vi "图像色彩识别.vi"() -> ()   [LabVIEW 2020]
uses:
  <vilib>/vision/NI_Vision_Development_Module.lvlib
panel:
  out "FoundYellow":bool
  out "FoundGreen":bool
  out "error out":errorcluster
  out "FoundRed":bool
  in  "停止":bool
  out "Color Spectrum":dbl[](array[numeric]) format="%.2f"
  in  "Rectangle":T1={"Left"=300, "Top"=170, "Right"=441, "Bottom"=320, "Rotation"=0.0} {"Rotation" min=-90.0 max=90.0 step=1.0 format="%.2f"; "Left" scale=0.0..1024.0; "Right" scale=0.0..1024.0}
  in  "File Path":path
  out "Image":T2(plugin-control)
  # "画框给出的左边值x,y格式给\n出，输入时注意对应"
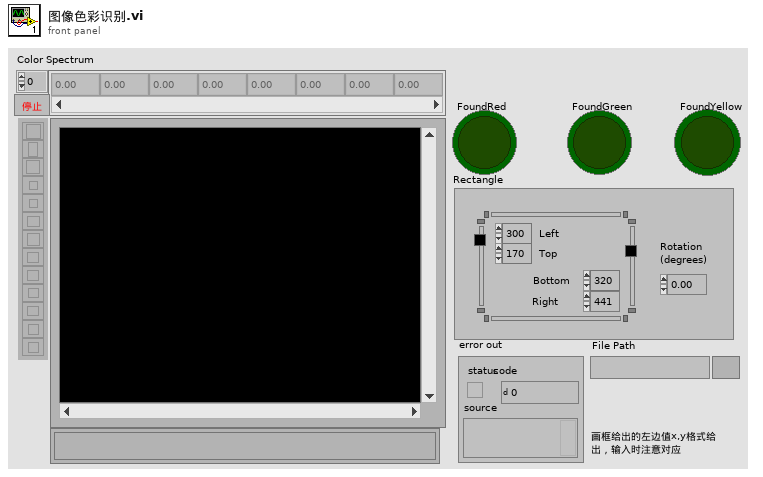
[diagram p1: front panel]
types:
  T1 = typedef "IMAQ Rectangle" = cluster{"Left":i32, "Top":i32, "Right":i32, "Bottom":i32, "Rotation":dbl}
  T2 = typedef "IMAQ Image.ctl" = refnum<image>
  T3 = typedef "ROI Descriptor" = cluster{"Global Rectangle":i32[], "Contours":cluster{"ID":enum32{"External", "Internal"}, "Type":u32, "Coordinates":i32[]}[]}
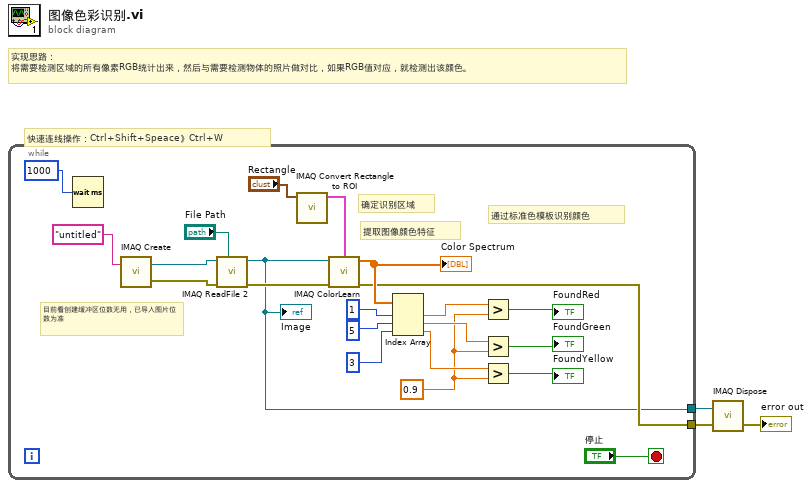
[diagram p0: block diagram]
diagram:
  # "快速连线操作：Ctrl+Shift+Speace》Ctrl+W"
  # "实现思路：\n将需要检测区域的所有像素RGB统计出来，然后与需要检测物体的照片做对比，如果RGB值对应，就检测出该颜色。"
  n1 = while {
    tunnel: [w13] -> w3
    tunnel: [w12] -> w2
    stop <- "停止" stop-if-true
    w4 = 0.9 ("y")
    # "通过标准色模板识别颜色"
    # "提取图像颜色特征"
    # "确定识别区域"
    # "目前看创建缓冲区位数无用，已导入图片位数为准"
    n2 = Wait (ms)(milliseconds to wait=u32 1000 ("等待时间（毫秒）")) -> ()  [unwired: 1 out]
    n3 = call "IMAQ Create"("Image Name"="untitled") -> ("New Image"=w14:T2, "error out"=w25:errorcluster)  [unwired: 4 in]
    n4 = call "IMAQ ReadFile 2"("File Path"="File Path", "error in (no error)"=w25, "Image"=w14) -> ("error out"=w24:errorcluster, "Image Out"=w12:T2)  [unwired: 4 in, 3 out]
    "Image" <- w12
    n5 = call "IMAQ Convert Rectangle to ROI"("Rectangle"="Rectangle") -> ("ROI Descriptor"=w21:T3)  [unwired: 8 in, 1 out]
    n6 = call "IMAQ ColorLearn"("ROI Descriptor"=w21, "Image"=w12, "error in (no error)"=w24) -> ("Color Spectrum"=w17:dbl[], "error out"=w13:errorcluster)  [unwired: 5 in]
    "Color Spectrum" <- w17
    n7 = Index Array(array=w17, index #1=1 ("索引"), index #2=5 ("索引"), index #3=3 ("索引")) -> (element #1=w9:dbl, element #2=w6:dbl, element #3=w5:dbl)
    n8 = Greater?(x=w9, y=w4) -> (0:→"FoundRed":bool)
    n9 = Greater?(x=w6, y=w4) -> (0:→"FoundGreen":bool)
    n10 = Greater?(x=w5, y=w4) -> (0:→"FoundYellow":bool)
  }
  n11 = call "IMAQ Dispose"("Image"=w2, "error in (no error)"=w3) -> ("error out"=→"error out":errorcluster)  [unwired: 4 in]
